vi "Parse Timestamp Array.vi"(6 "Seperator":string=",", 8 "error in":errorcluster, 9 "Input":string, 10 "csv string":string, 11 "Named Columns Parser in":refnum<class "Named Fields Parser.lvclass">) -> (0 "error out":errorcluster, 2 "Timestamp Array":timestamp[](array[timestamp]) format="%<%x %.3X>T", 3 "Named Columns Parser out":refnum<class "Named Fields Parser.lvclass">)   [LabVIEW 2020, in "Named Fields Parser.lvclass"]
uses:
  Named Fields Parser.lvclass
  Named Fields Parser.lvclass/Named Fields Parser.ctl
  38260a8c-1a19-4655-b4da-4e8077795298.vi
  7a224f0f-72cb-46f0-b414-9ad9b5680fe1.vi
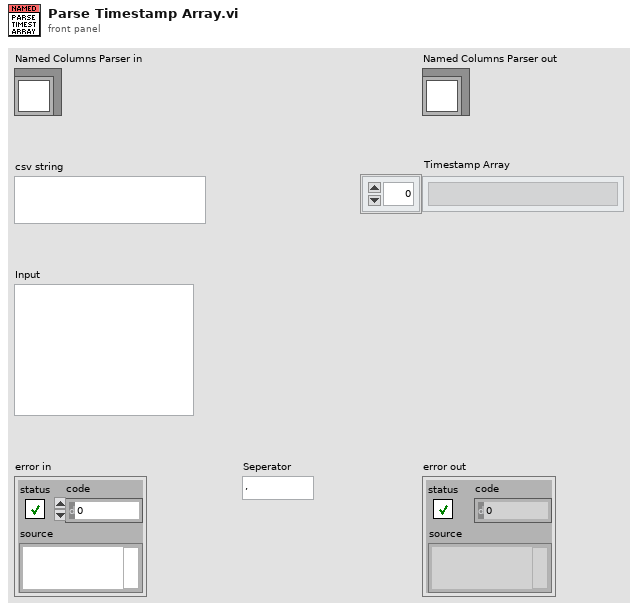
[diagram p1: front panel]
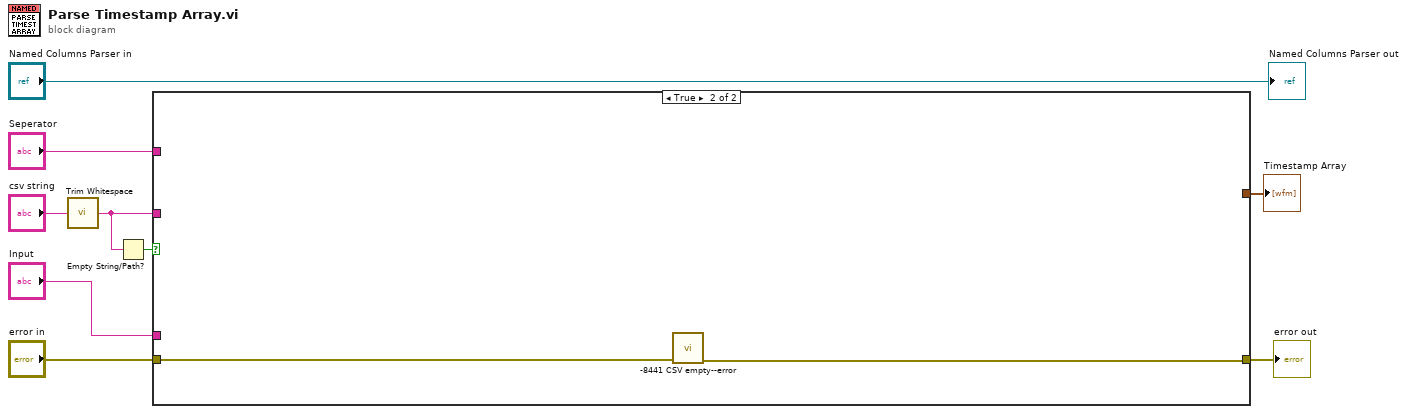
[diagram p0: block diagram]
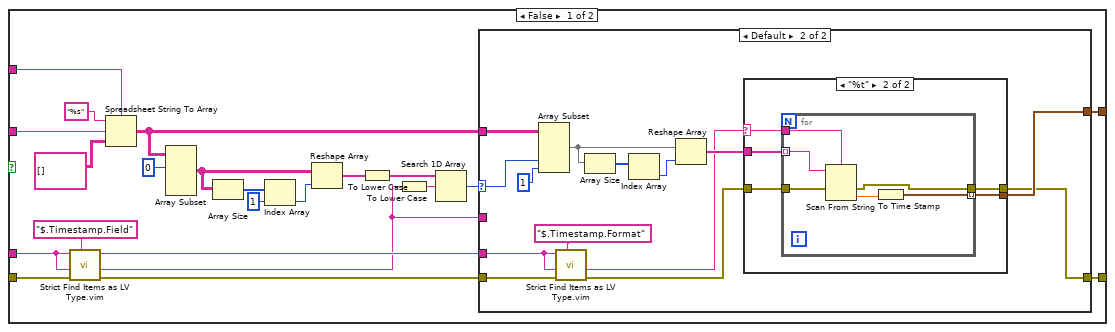
[diagram p2: hidden frame]
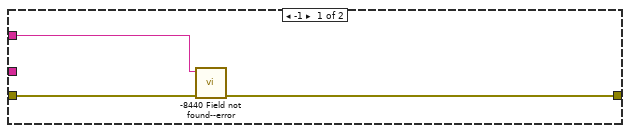
[diagram p3: hidden frame]
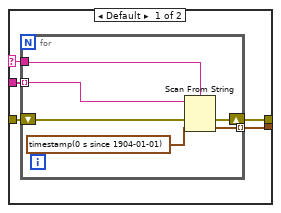
[diagram p4: hidden frame]
diagram:
  n1 = call <vilib>:"Trim Whitespace.vi"("string"="csv string") -> ("trimmed string"=w1:string)  [unwired: 1 in]
  n2 = Empty String/Path?(string/path=w1) -> (empty?=w3:bool)
  n3 = case shown="True" w3 {
    tunnel: "error in" -> [w29 w72]
    tunnel: w1 -> [w26 _]
    tunnel: [w25 _] -> w7
    tunnel: [w24 w71] -> w6
    tunnel: "Seperator" -> [w23 _]
    tunnel: "Input" -> [w22 _]
    frame False {
      n4 = call "Strict Find Items as LV Type.vim"("$Path or Item Name"="$.Timestamp.Field", "error in"=w29, "Data Type and Default Value"=w22, "<JSON>"=w22) -> ("error out"=w27:errorcluster, "Data out"=w12:string, "<JSON> dup"=w14:string)  [unwired: 5 in]
      n5 = Spreadsheet String To Array(delimiter (Tab)=w23, format string="%s", spreadsheet string=w26, array type (2D Dbl)=string[][] []) -> (array=w21:string[][])
      n6 = Array Subset(array=w21, index (row)=0 ("index")) -> (w16:string[][])  [unwired: 3 in]
      n7 = Array Size(array=w16) -> (size(s)=w19:i32[])
      n8 = Index Array(array=w19, index=1) -> (element=w17:i32)
      n9 = Reshape Array(w16, w17) -> (w15:string[])
      n10 = To Lower Case(string=w15) -> (all lower case string=w11:string[])
      n11 = To Lower Case(string=w12) -> (all lower case string=w10:string)
      n12 = Search 1D Array(1D array=w11, element=w10) -> (index of element=w13:i32)  [unwired: 1 in]
      n13 = case shown="Default" w13 {
        selector: w13 -> [_ w36]
        tunnel: w27 -> [w34 w42]
        tunnel: [_ w40] -> w25
        tunnel: [w33 w39] -> w24
        tunnel: w21 -> [_ w38]
        tunnel: w14 -> [_ w37]
        tunnel: w12 -> [w32 _]
        frame -1 {
          n14 = call "-8440 Field not found--error.vi"("error in"=w34, "Field Name"=w32) -> ("error out"=w33:errorcluster)  [unwired: 9 in]
        }
        frame Default {
          n15 = Array Subset(array=w38, index (col)=w36, length (col)=1 ("length")) -> (w47:string[][])  [unwired: 2 in]
          n16 = call "Strict Find Items as LV Type.vim"("$Path or Item Name"="$.Timestamp.Format", "error in"=w42, "Data Type and Default Value"=w37, "<JSON>"=w37) -> ("error out"=w44:errorcluster, "Data out"=w41:string)  [unwired: 5 in, 1 out]
          n17 = Array Size(array=w47) -> (size(s)=w48:i32[])
          n18 = Index Array(array=w48) -> (element=w46:i32)  [unwired: 1 in]
          n19 = Reshape Array(w47, w46) -> (w45:string[])
          n20 = case shown="\"%t\"" w41 {
            selector: w41 -> [w51 w63]
            tunnel: w45 -> [w53 w62]
            tunnel: w44 -> [w52 w64]
            tunnel: [w50 w61] -> w40
            tunnel: [w49 w60] -> w39
            frame Default {
              n21 = for {
                tunnel: w51 -> [w59]
                shift-right: [w57] -> w49
                shift-left: w52 -> [w58]
                tunnel: w53 -> [w56] mode=indexing
                tunnel: [w55] -> w50 mode=indexing
                n22 = Scan From String(format string=w59, input string=w56, error in=w58, default 1=timestamp(0 s since 1904-01-01) ("Time Stamp")) -> (error out=w57:errorcluster, output 1=w55:timestamp)  [unwired: 1 in, 2 out]
              }
            }
            frame "%t" {
              n23 = for {
                tunnel: w64 -> [w70]
                tunnel: w63 -> [w69]
                tunnel: w62 -> [w68] mode=indexing
                tunnel: [w66] -> w61 mode=indexing
                tunnel: [w65] -> w60
                n24 = Scan From String(format string=w69, input string=w68, error in=w70) -> (error out=w65:errorcluster, output 1=w67:dbl)  [unwired: 2 in, 2 out]
                n25 = To Time Stamp(1:w67) -> (0:w66:timestamp)
              }
            }
          }
        }
      }
    }
    frame True {
      n26 = call "-8441 CSV empty--error.vi"("error in"=w72) -> ("error out"=w71:errorcluster)  [unwired: 10 in]
    }
  }
  "error out" <- w6
  "Timestamp Array" <- w7
  "Named Columns Parser out" <- "Named Columns Parser in"
